vi "Day09-2.vi"() -> ()   [LabVIEW 2021]
uses:
  e8067021-3399-4566-9da4-0f30890c607a.vi
  1fa128aa-b721-40bb-8710-f8c80fc8b9e9.vi
  <vilib>/Comparison/Less/Less Functor/Less Functor.lvclass
panel:
  out "product":i32
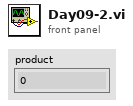
[diagram p1: front panel]
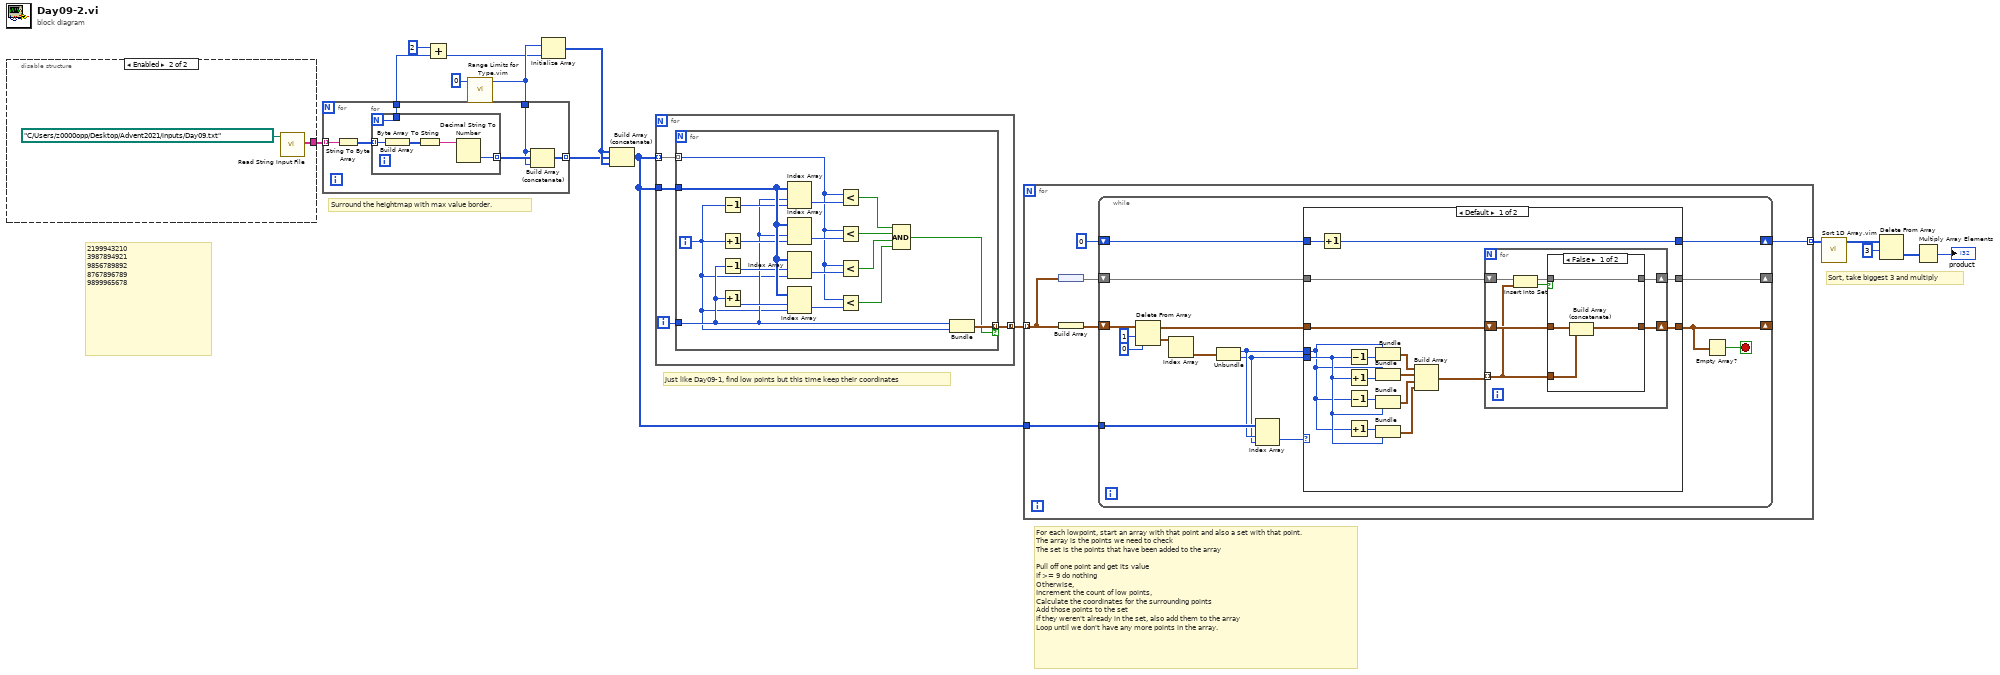
[diagram p0: block diagram]
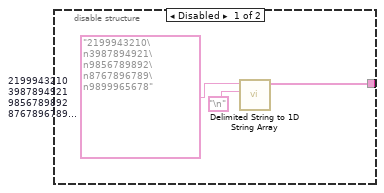
[diagram p4: hidden frame]
diagram:
  # "For each lowpoint, start an array with that point and also a set with that point.\nThe array is the points we need to check\nThe set is the points that have been added to the array\n\nPull off one point and get its value\nIf >= 9 do nothing\nOtherwise,\nIncrement the count of low points,\nCalculate the coordinates for the surrounding points\nAdd those points to the set\nIf they weren't already in the set, also add them to the array\nLoop until we don't have any more points in the array."
  # "Sort, take biggest 3 and multiply"
  # "Just like Day09-1, find low points but this time keep their coordinates"
  # "2199943210\n3987894921\n9856789892\n8767896789\n9899965678"
  # "Surround the heightmap with max value border."
  n1 = disable-structure shown="Enabled" {
    disable-tunnel: [w16 w19] -> w15
    frame Disabled {
      w18 = "2199943210\n3987894921\n9856789892\n8767896789\n9899965678"  # 2199943210 3987894921 9856789892 8767896789 9899965678
      n2 = call <vilib>:"Delimited String to 1D String Array.vi"("delimiter"="\n", "delimited string"=w18) -> ("string array"=w16:string[])  [unwired: 9 in]
    }
    frame Enabled {
      n3 = call "Read String Input File.vi"("file path (dialog if empty)"=path "C:/Users/z0000opp/Desktop/Advent2021/inputs/Day09.txt") -> ("input values"=w19:string[])  [unwired: 10 in]
    }
  }
  n4 = call "Range Limits for Type.vim"("type"=0) -> ("maximum value for type"=w13:i32)  [unwired: 9 in, 1 out]
  n5 = for {
    tunnel: w15 -> [w26] mode=indexing
    tunnel: [w22] -> w8 mode=indexing
    tunnel: w13 -> [w23]
    tunnel: [w21] -> w12
    n6 = String To Byte Array(string=w26) -> (unsigned byte array=w25:u8[])
    n7 = for {
      N -> [w27]
      tunnel: w25 -> [w31] mode=indexing
      tunnel: [w28] -> w24 mode=indexing
      tunnel: [w27] -> w21
      n8 = Build Array(w31) -> (w30:u8[])
      n9 = Byte Array To String(unsigned byte array=w30) -> (string=w29:string)
      n10 = Decimal String To Number(string=w29) -> (number=w28:i32)  [unwired: 2 in, 1 out]
    }
    n11 = Build Array (concatenate)(w23, w24, w23) -> (w22:i32[])
  }
  n12 = Add(x=2, y=w12) -> (x+y=w11:i32)
  n13 = Initialize Array(w13, w11) -> (w9:i32[])
  n14 = Build Array (concatenate)(w9, w8, w9) -> (w6:i32[][])
  n15 = for {
    tunnel: w6 -> [w35] mode=indexing
    tunnel: w6 -> [w34]
    tunnel: [w32] -> w7 mode=concatenating
    i -> [w33]
    n16 = for {
      tunnel: w35 -> [w40] mode=indexing
      tunnel: w34 -> [w53]
      tunnel: w33 -> [w39]
      tunnel: [w37] -> w32 mode=indexing if=w36
      i -> [w38]
      n17 = Decrement(x=w38) -> (x-1=w52:i32)
      n18 = Increment(x=w38) -> (x+1=w51:i32)
      n19 = Decrement(x=w39) -> (x-1=w50:i32)
      n20 = Increment(x=w39) -> (x+1=w49:i32)
      n21 = Index Array(array=w53, index (row)=w39, index (col)=w52) -> (element=w48:i32)
      n22 = Index Array(array=w53, index (row)=w39, index (col)=w51) -> (element=w47:i32)
      n23 = Index Array(array=w53, index (row)=w50, index (col)=w38) -> (element=w46:i32)
      n24 = Index Array(array=w53, index (row)=w49, index (col)=w38) -> (element=w45:i32)
      n25 = Less?(x=w40, y=w48) -> (x < y?=w44:bool)
      n26 = Less?(x=w40, y=w47) -> (x < y?=w43:bool)
      n27 = Less?(x=w40, y=w46) -> (x < y?=w42:bool)
      n28 = Less?(x=w40, y=w45) -> (x < y?=w41:bool)
      n29 = Compound Arithmetic op=AND(w44, w43, w42, w41) -> (w36:bool)
      n30 = Bundle(w39, w38) -> (w37:cluster{i32, i32})  [unwired: 1 in]
    }
  }
  n31 = for {
    tunnel: w7 -> [w55] mode=indexing
    tunnel: w6 -> [w59]
    tunnel: [w56] -> w5 mode=indexing
    n32 = node(w55) -> (w54:set{cluster{i32, i32}})
    n33 = Build Array(w55) -> (w58:cluster{i32, i32}[])
    n34 = while {
      tunnel: w59 -> [w71]
      shift-right: [w66] -> _
      shift-left: w58 -> [w75]
      shift-right: [w68] -> w56
      shift-left: 0 -> [w69]
      shift-right: [w62] -> _
      shift-left: w54 -> [w60]
      stop <- w65 stop-if-true
      n35 = Delete From Array(array=w75, length=1, index=0) -> (deleted portion=w72:cluster{i32, i32}[], array with subset deleted=w67:cluster{i32, i32}[])
      n36 = Index Array(array=w72) -> (element=w61:cluster{i32, i32})  [unwired: 1 in]
      n37 = Unbundle(w61) -> (w64:i32, w63:i32)
      n38 = Index Array(array=w71, index (row)=w64, index (col)=w63) -> (element=w70:i32)
      n39 = case shown="Default" w70 {
        tunnel: w69 -> [w92 w108]
        tunnel: [w91 w108] -> w68
        tunnel: w67 -> [w88 w107]
        tunnel: [w86 w107] -> w66
        tunnel: w64 -> [w80 _]
        tunnel: w63 -> [w82 _]
        tunnel: w60 -> [w76 w106]
        tunnel: [w77 w106] -> w62
        frame Default {
          n40 = Increment(x=w92) -> (x+1=w91:i32)
          n41 = Decrement(x=w82) -> (x-1=w83:i32)
          n42 = Increment(x=w82) -> (x+1=w81:i32)
          n43 = Decrement(x=w80) -> (x-1=w79:i32)
          n44 = Increment(x=w80) -> (x+1=w78:i32)
          n45 = Bundle(w80, w83) -> (w90:cluster{i32, i32})  [unwired: 1 in]
          n46 = Bundle(w80, w81) -> (w89:cluster{i32, i32})  [unwired: 1 in]
          n47 = Bundle(w79, w82) -> (w84:cluster{i32, i32})  [unwired: 1 in]
          n48 = Bundle(w78, w82) -> (w85:cluster{i32, i32})  [unwired: 1 in]
          n49 = Build Array(w90, w89, w84, w85) -> (w87:cluster{i32, i32}[])
          n50 = for {
            tunnel: w87 -> [w95] mode=indexing
            shift-right: [w98] -> w86
            shift-left: w88 -> [w99]
            shift-right: [w97] -> w77
            shift-left: w76 -> [w94]
            n51 = Insert Into Set(10:w95, 11:w94) -> (2:w96:bool, 3:w93:set{cluster{i32, i32}})
            n52 = case shown="False" w96 {
              tunnel: w99 -> [w103 w105]
              tunnel: [w102 w105] -> w98
              tunnel: w95 -> [w101 _]
              tunnel: w93 -> [w100 w104]
              tunnel: [w100 w104] -> w97
              frame False {
                n53 = Build Array (concatenate)(w103, w101) -> (w102:cluster{i32, i32}[])
              }
              frame True {
              }
            }
          }
        }
        frame 9.. {
        }
      }
      n54 = Empty Array?(array=w66) -> (empty?=w65:bool)
    }
  }
  n55 = call "Sort 1D Array.vim"("unsorted array"=w5) -> ("sorted array"=w4:i32[])  [unwired: 10 in]
  n56 = Delete From Array(array=w4, length=3) -> (deleted portion=w2:i32[])  [unwired: 1 in, 1 out]
  n57 = Multiply Array Elements(1:w2) -> (0:→"product":i32)
